vi "JSONRPC-RIPDispatcher.vi"(8 "error in":errorcluster, 11 "input string":string) -> (0 "error out":errorcluster, 3 "response":string)   [LabVIEW 2020]
doc: "Parse a JSONRPC 2.0 string and invokes the corresponding method."
panel:
  # "RIPDispatcher"
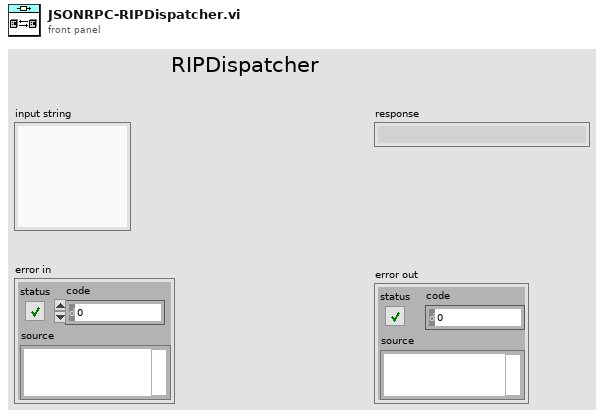
[diagram p1: front panel]
types:
  T1 = cluster{"params":string, "id":string, "method":enum16{"open", "close", "start", "stop", "get", "set", "info", "UNDEFINED"}}
  T2 = enum16{"open", "close", "start", "stop", "get", "set", "info", "UNDEFINED"}
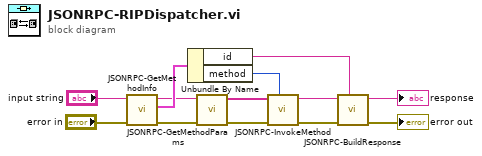
[diagram p0: block diagram]
diagram:
  n1 = call "JSONRPC-GetMethodInfo.vi"("error in"="error in", "input string"="input string") -> ("error out"=w11:errorcluster, "RPC"=w5:T1, "input string"=w3:string)  [unwired: 7 in]
  n2 = Unbundle By Name(w5) -> ("id"=w4:string, "method"=w1:T2)
  n3 = call "JSONRPC-GetMethodParams.vi"("error in"=w11, "input string"=w3) -> ("error out"=w10:errorcluster, "params"=w9:string[])  [unwired: 8 in]
  n4 = call "JSONRPC-InvokeMethod.vi"("method"=w1, "error in (no error)"=w10, "params"=w9) -> ("error out"=w13:errorcluster, "result"=w8:string)  [unwired: 6 in, 1 out]
  n5 = call "JSONRPC-BuildResponse.vi"("ID"=w4, "error in"=w13, "Result"=w8) -> ("error out"=→"error out":errorcluster, "JSONRPC Response"=→"response":string)  [unwired: 7 in]
